vi "oscilloscopio.vi"() -> ()   [LabVIEW 2018]
panel:
  out "Frequenza":dbl format="%#_6f"
  in  "isteresi":dbl=0.7 min=0.0 max=2.0 step=0.1
  in  "livello":dbl=1.0 min=0.0 step=0.5
  in  "% trigger":dbl(slide) min=0.0 max=100.0 step=10.0 scale=0.0..100.0
  in  "?":bool
  out "Rms Ch 2":dbl=1.41340783379716 format="%.3f"
  out "Rms Ch 1":dbl=2.1208739363094185 format="%.3f"
  out "S P.Apparente":dbl=2.997659836075951 format="%.3f"
  out "Q P.Reattiva":dbl=2.1196030662964884 format="%.3f"
  out "P attiva":dbl=2.1197281274185666 format="%.3f"
  in  "?":bool=TRUE
  in  "s/Div":dbl(ring)=0.01 items=["100ms"=0.1, "50ms"=0.05, "20ms"=0.02, "10ms"=0.01, "5ms"=0.005, "2ms"=0.002, "1ms"=0.001]
  in  "Volt/Div Ch 2":dbl(ring)=1.0 items=["10V"=10.0, "5V"=5.0, "2V"=2.0, "1V"=1.0, "500mV"=0.5, "200mV"=0.2, "100mV"=0.1, "50mV"=0.05, "20mV"=0.02, "10mV"=0.01]
  in  "Volt/Div Ch 1":dbl(ring)=1.0 items=["10V"=10.0, "5V"=5.0, "2V"=2.0, "1V"=1.0, "500mV"=0.5, "200mV"=0.2, "100mV"=0.1, "50mV"=0.05, "20mV"=0.02, "10mV"=0.01]
  in  "scelta":bool
  out "?":waveform(dbl)[](graph)=[{"t0"=timestamp(62.4 s since 1904-01-01), "dt"=0.0001, "Y"=array[1000 elements]}, {"t0"=timestamp(62.4 s since 1904-01-01), "dt"=0.0001, "Y"=array[1000 elements]}]
  out "ultimo trigger":i32=995
  out "1 Trigger":i32=195
  out "valore di picco   2":dbl=2.014596205172248
  out "valore di picco":dbl=3.0180810106073213
  in  "N":dbl=1000.0 min=2.0 step=100.0
  # "TRIGGER"
  # "SCELTA"
  # "HORIZONTAL"
  # "MODALITY"
  # "VERTICAL"
  # "salita"
  # "discesa"
  # "Ch 1"
  # "Ch 2"
  # "Ch 2"
  # "Ch 1"
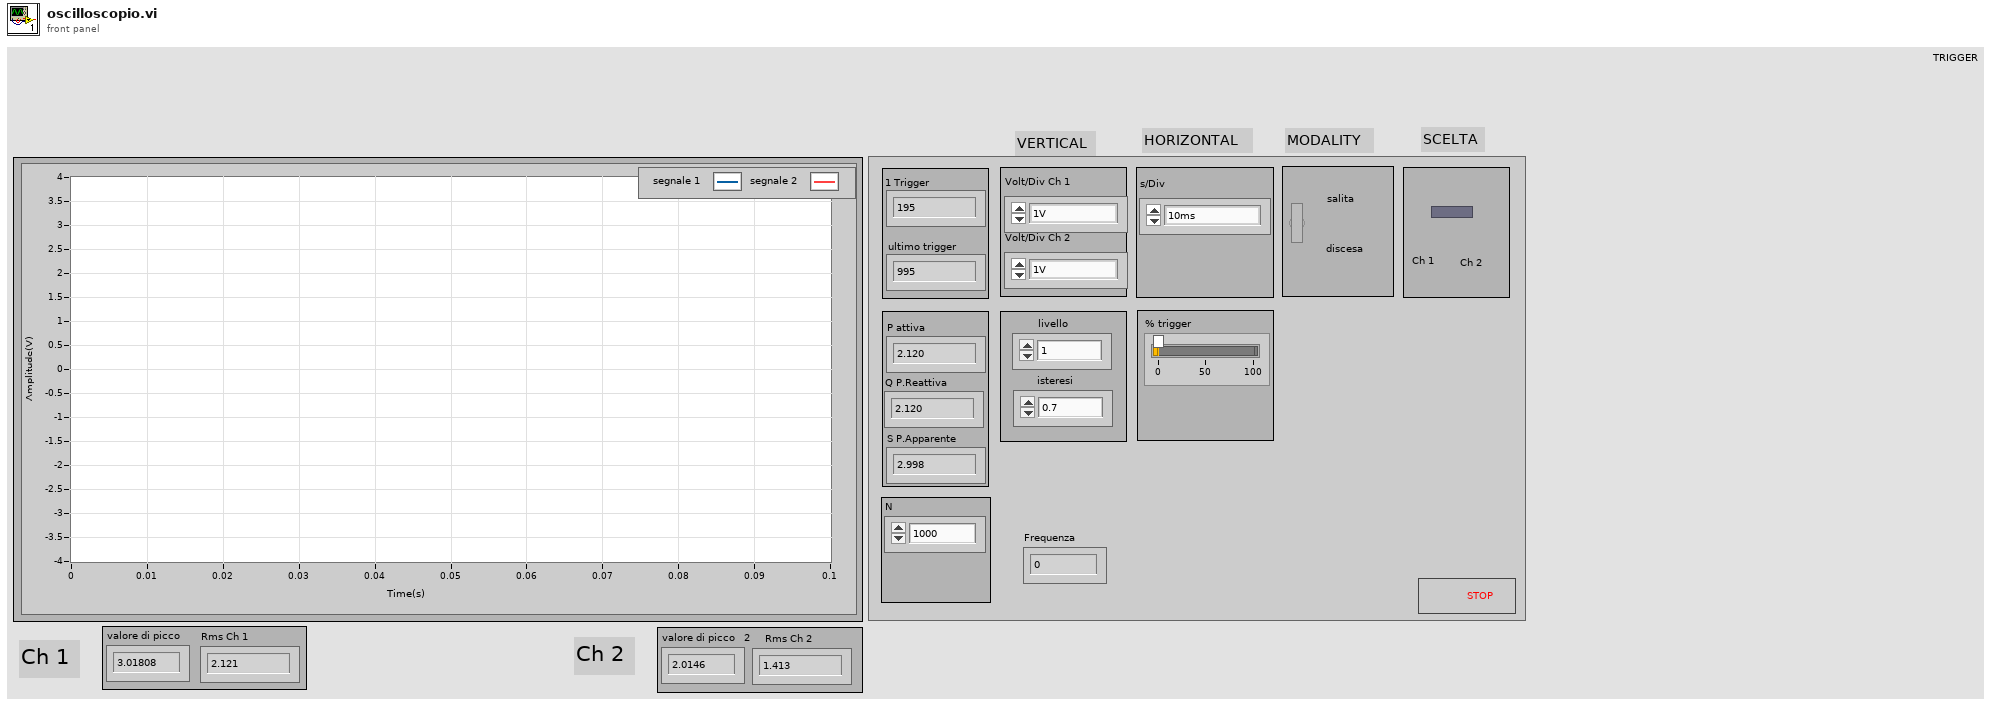
[diagram p1: front panel]
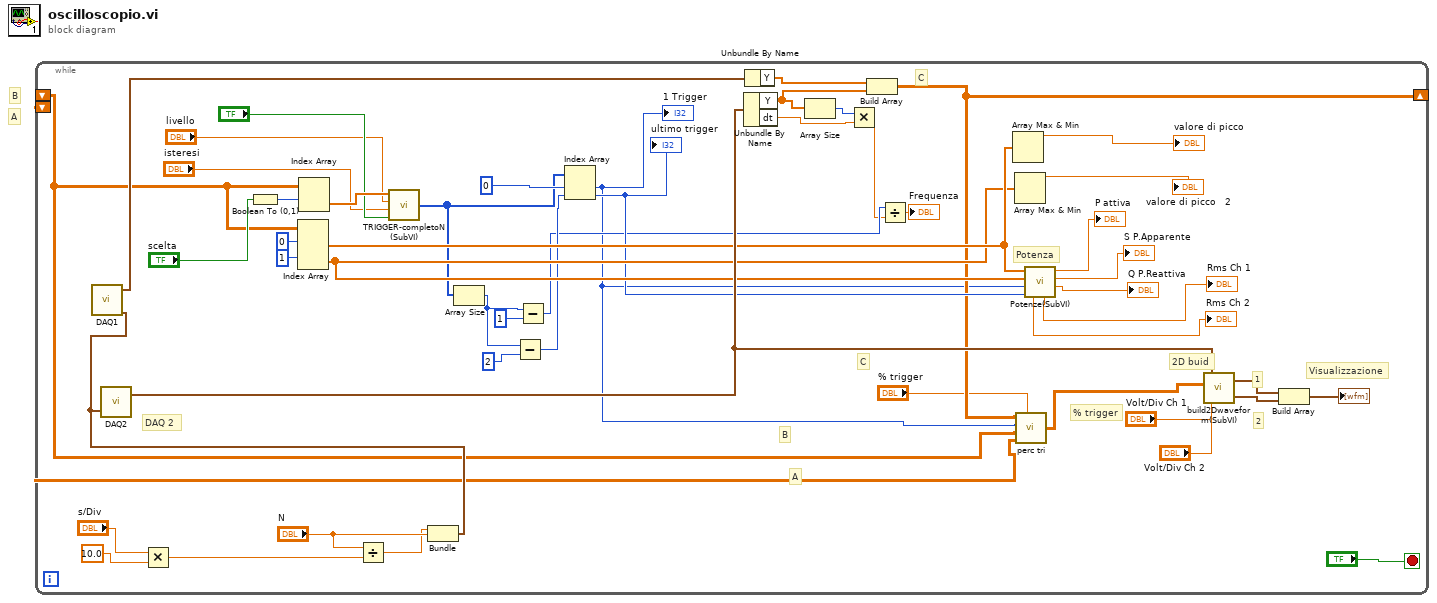
[diagram p0: block diagram]
diagram:
  # "A"
  # "B"
  n1 = while {
    shift-right: [w5] -> _
    shift-left: _ -> [w3]
    shift-left: _ -> [w2]
    stop <- "?" stop-if-true
    # "Visualizzazione"
    # "2"
    # "1"
    # "Potenza"
    # "DAQ 2"
    # "2D buid"
    # "% trigger"
    # "B"
    # "A"
    # "C"
    # "C"
    n2 = Multiply(x="s/Div", y=10.0) -> (x*y=w18:dbl)
    n3 = Boolean To (0,1)(Boolean="scelta") -> (0, 1=w50:i16)
    n4 = Index Array(array=w3, index (row) #1=0 ("index (row)"), index (row) #2=1 ("index (row)")) -> (element #1=w28:dbl[], element #2=w27:dbl[])  [unwired: 2 in]
    n5 = Index Array(array=w3, index (row)=w50) -> (element=w49:dbl[])  [unwired: 1 in]
    n6 = Divide(x="N", y=w18) -> (x/y=w15:dbl)
    n7 = call "TRIGGER-completoN (SubVI).vi"("Modalità"="?", "isteresi"="isteresi", "livello"="livello", "Segnale B"=w49) -> ("eventi di trigger"=w16:i32[])
    n8 = Bundle(w15, "N"="N") -> (w41:cluster{dbl, "N":dbl})  [unwired: 1 in]
    n9 = call "DAQ1.vi"("sampling info"=w41) -> ("Waveform"=w44:waveform(dbl))  [unwired: 5 in]
    n10 = call "DAQ2.vi"("sampling info"=w41) -> ("Waveform"=w42:waveform(dbl))  [unwired: 3 in]
    n11 = Array Size(array=w16) -> (size(s)=w11:i32)
    n12 = Subtract(x=w11, y=2) -> (x-y=w19:i32)
    n13 = Subtract(x=w11, y=1) -> (x-y=w9:i32)
    n14 = Index Array(array=w16, index #1=0 ("index"), index #2=w19) -> (element #1=w4:i32, element #2=w17:i32)
    "1 Trigger" <- w4
    "ultimo trigger" <- w17
    n15 = Unbundle By Name(w42) -> ("Y"=w14:dbl[], "dt"=w12:dbl)
    n16 = Unbundle By Name(w44) -> ("Y"=w43:dbl[])
    n17 = Array Size(array=w14) -> (size(s)=w13:i32)
    n18 = Multiply(x=w13, y=w12) -> (x*y=w8:dbl)
    n19 = Build Array(w43, w14) -> (w5:dbl[][])
    n20 = Divide(x=w9, y=w8) -> (x/y=→"Frequenza":dbl)
    n21 = Array Max & Min(array=w28) -> (max value=→"valore di picco":dbl)  [unwired: 3 out]
    n22 = Array Max & Min(array=w27) -> (max value=→"valore di picco   2":dbl)  [unwired: 3 out]
    n23 = call "perc tri.vi"("C"=w5, "trigger"=w4, "B"=w3, "A"=w2, "%"="% trigger") -> ("Array"=w6:dbl[][])
    n24 = call "Potenze(SubVI).vi"("ultimo trigger"=w17, "1 trigger"=w4, "2"=w27, "1"=w28) -> ("Q P.Reattiva"=→"Q P.Reattiva":dbl, "S P.Apparente"=→"S P.Apparente":dbl, "P attiva"=→"P attiva":dbl, "Rms Ch 1"=→"Rms Ch 1":dbl, "Rms Ch 2"=→"Rms Ch 2":dbl)  [unwired: 3 in]
    n25 = call "build2Dwaveform(SubVI).vi"("Volt/Div Ch 2"="Volt/Div Ch 2", "Volt/Div Ch 1"="Volt/Div Ch 1", "Array"=w6, "waveform"=w42) -> ("secondo segnale"=w45:waveform(dbl), "primo segnale"=w46:waveform(dbl))
    n26 = Build Array(w46, w45) -> (→"?":waveform(dbl)[])
  }
